vi "my_onnx_test.vi"() -> ()   [LabVIEW 2022 SP3]
panel:
  out "error out load":errorcluster
  out "error out object":errorcluster
  out "appended path":path
  out "millisecond timer value":u32
  in  "OK Button":bool
  in  "关闭界面":bool
  in  "图片名":string
  out "模型名":string="deeplabv3_resnet101.onnx"
  out "error out":errorcluster
  out "程序路径名":path
  out "return value":i32
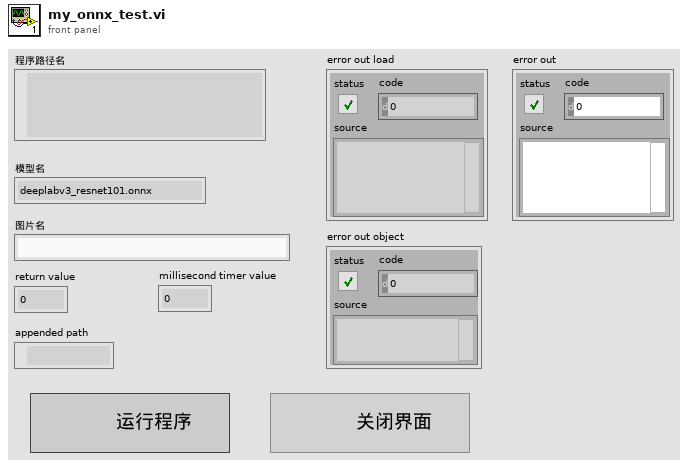
[diagram p1: front panel]
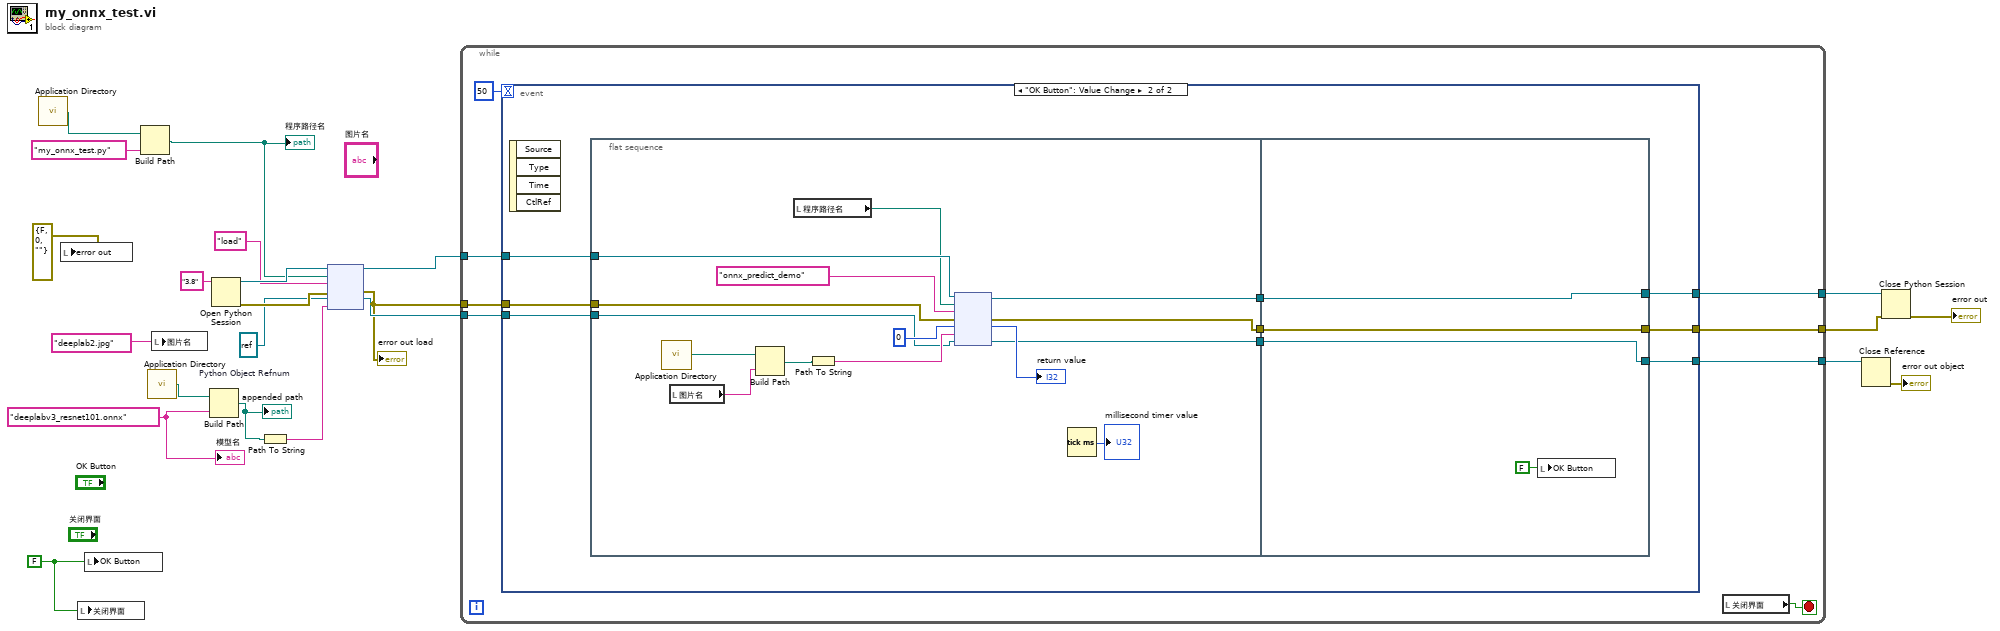
[diagram p0: block diagram]
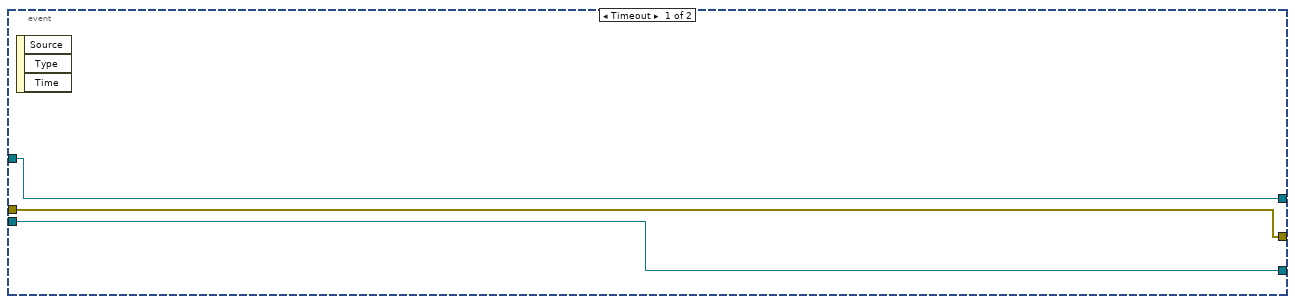
[diagram p2: hidden frame]
diagram:
  w7 = refnum<k38> refnum  # Python Object Refnum
  w14 = "deeplabv3_resnet101.onnx"
  w21 = FALSE ("OK Button")
  n1 = call <vilib>:"Application Directory.vi"() -> ("Application Directory"=w3:path)
  n2 = local write "error out"(errorcluster {"status"=FALSE, "code"=0, "source"=""} ("error out")) -> ()
  n3 = local write "关闭界面"(w21) -> ()
  n4 = local write "OK Button"(w21) -> ()
  n5 = Build Path(base path=w3, name or relative path="my_onnx_test.py") -> (appended path=w11:path)
  "程序路径名" <- w11
  n6 = call <vilib>:"Application Directory.vi"() -> ("Application Directory"=w16:path)
  n7 = local write "图片名"("deeplab2.jpg") -> ()
  n8 = Build Path(base path=w16, name or relative path=w14) -> (appended path=w15:path)
  "appended path" <- w15
  n9 = Open Python Session(python version="3.8" ("Python version")) -> (session out=w12:refnum<k35>, error out=w9:errorcluster)  [unwired: 2 in]
  n10 = Path To String(path=w15) -> (string=w8:string)
  n11 = node(w12, w11, "load" ("function name"), w9, w7, w8) -> (w4:refnum<k35>, w5:errorcluster, w6:refnum<k38>)  [unwired: 1 in, 2 out]
  "error out load" <- w5
  n12 = while {
    tunnel: w4 -> [w29]
    tunnel: [w28] -> w18
    tunnel: [w27] -> w17
    tunnel: w5 -> [w26]
    tunnel: w6 -> [w25]
    tunnel: [w24] -> w2
    stop <- w31 stop-if-true
    n13 = event shown="[1] \"OK Button\": Value Change" {
      selector: _ -> [_ _]
      dyn-events: _ -> [_ _]
      timeout: 50 -> [_ _]
      tunnel: w29 -> [w34 w43]
      tunnel: [w34 w42] -> w28
      tunnel: [w33 w40] -> w27
      tunnel: w26 -> [w33 w38]
      tunnel: w25 -> [w32 w37]
      tunnel: [w32 w36] -> w24
      event Timeout {
        n14 = event-data() -> ()  [unwired: 1 in, 3 out]
      }
      event "OK Button": Value Change {
        n15 = event-data() -> ()  [unwired: 1 in, 4 out]
        n16 = flat-sequence {
          tunnel: w43 -> [w53]
          tunnel: [w51] -> w41
          tunnel: [w50] -> w39
          tunnel: w38 -> [w49]
          tunnel: w37 -> [w47]
          tunnel: [w44] -> w35
          tunnel: [w61] -> w42
          tunnel: w41 -> [w61]
          tunnel: [w60] -> w40
          tunnel: w39 -> [w60]
          tunnel: [w59] -> w36
          tunnel: w35 -> [w59]
          frame #0 {
            n17 = call <vilib>:"Application Directory.vi"() -> ("Application Directory"=w45:path)
            n18 = local read "图片名"() -> (w58:string)
            n19 = Build Path(base path=w45, name or relative path=w58) -> (appended path=w56:path)
            n20 = local read "程序路径名"() -> (w48:path)
            n21 = Path To String(path=w56) -> (string=w57:string)
            n22 = node(w53, w48, "onnx_predict_demo" ("function name"), w49, 0, w57, w47) -> (w51:refnum<k35>, w50:errorcluster, →"return value":i32, w44:refnum<k38>)  [unwired: 1 in, 2 out]
            n23 = Tick Count (ms)() -> (millisecond timer value=→"millisecond timer value":u32)
          }
          frame #1 {
            n24 = local write "OK Button"(FALSE ("OK Button")) -> ()
          }
        }
      }
    }
    n25 = local read "关闭界面"() -> (w31:bool)
  }
  n26 = Close Reference(reference=w2) -> (error out=→"error out object":errorcluster)  [unwired: 1 in]
  n27 = Close Python Session(session in=w18, error in=w17) -> (11:→"error out":errorcluster)
  "模型名" <- w14
